vi "I32 1D to Data Type.vi"(8 "error in (no error)":errorcluster, 11 "I32 1D":i32[](array[numeric])) -> (0 "error out":errorcluster, 3 "Boolean out":refnum<class "I32 1D.lvclass">)   [LabVIEW 2017, in "I32 1D.lvclass"]
uses:
  <vilib>/gpm_packages/@cs/data-type-serializer/source/I32 1D/I32 1D.lvclass
  <vilib>/gpm_packages/@cs/data-type-serializer/source/I32 1D/I32 1D.lvclass/I32 1D.ctl
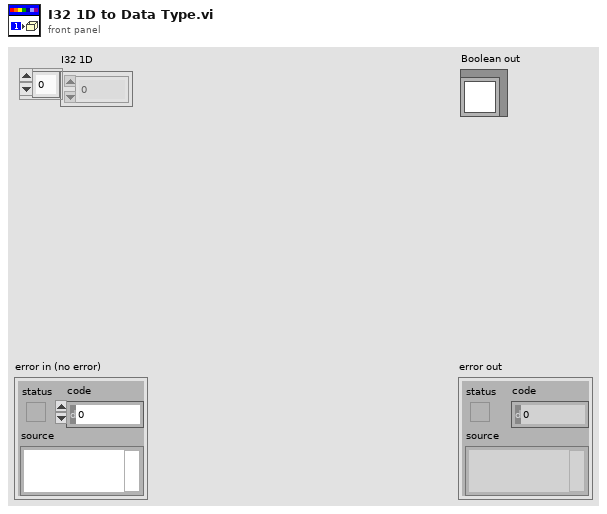
[diagram p1: front panel]
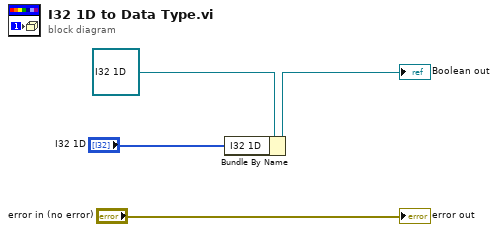
[diagram p0: block diagram]
diagram:
  n1 = Bundle By Name(cluster=refnum<class "I32 1D.lvclass"> refnum ("Boolean in"), "I32 1D"="I32 1D") -> (→"Boolean out":refnum<class "I32 1D.lvclass">)
  "error out" <- "error in (no error)"
